vi "lsig1.vi"(3 "x":u32) -> (1 "lsig1":u32)   [LabVIEW 2020, in "NI_SHA-256.lvclass"]
doc: "Computes the SHA-2 \\sigma_1(x) function."
uses:
  <vilib>/security/Message Digest/SHA-2/SHA-256/NI_SHA-256.lvclass
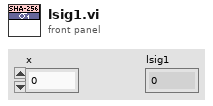
[diagram p1: front panel]
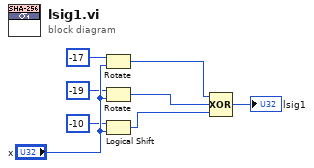
[diagram p0: block diagram]
diagram:
  n1 = Rotate(1:"x", 2:i16 -17 ("y")) -> (0:w1:u32)
  n2 = Rotate(1:"x", 2:i16 -19 ("y")) -> (0:w2:u32)
  n3 = Logical Shift(y=i16 -10, x="x") -> (x << y=w3:u32)
  n4 = Compound Arithmetic op=XOR(w1, w2, w3) -> (→"lsig1":u32)
